vi "Get Speed.vi"(8 "error in (no error)":errorcluster, 11 "Motor in":refnum<class "Motor.lvclass">) -> (0 "error out":errorcluster, 2 "Speed":dbl, 3 "Motor out":refnum<class "Motor.lvclass">)   [LabVIEW 2019, in "Motor.lvclass"]
uses:
  Motor.lvclass
  Motor.lvclass/Motor.ctl
  Motor Serial class/Serial.lvclass
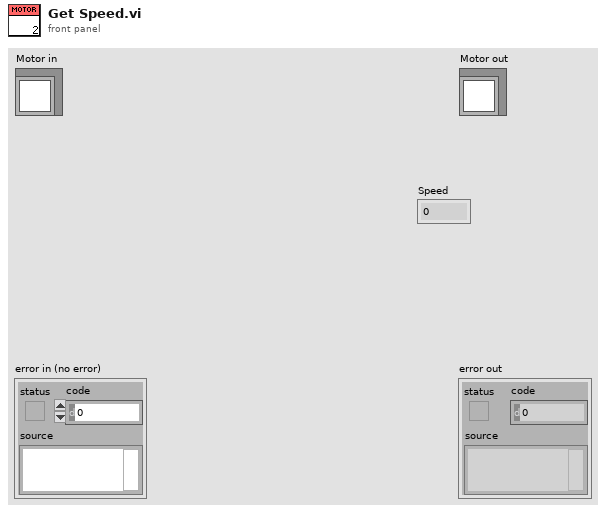
[diagram p1: front panel]
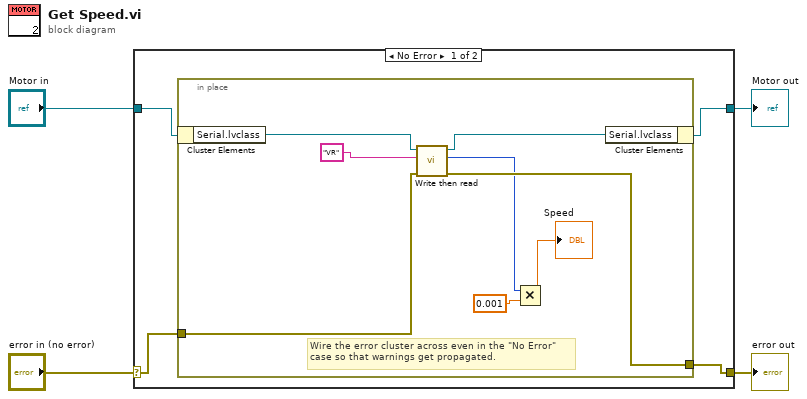
[diagram p0: block diagram]
diagram:
  n1 = case shown="No Error" "error in (no error)" {
    selector: "error in (no error)" -> [w5 w18]
    tunnel: [w6 w18] -> w3
    tunnel: [w7 w17] -> w1
    tunnel: "Motor in" -> [w8 w17]
    frame No Error {
      n2 = in-place {
        in-place-border: [w12] -> w6
        in-place-border: w5 -> [w13]
        # "Wire the error cluster across even in the \"No Error\"\ncase so that warnings get propagated."
        n3 = in-place-cluster #1(w8) -> ("Serial.lvclass"=w16:refnum<class "Serial.lvclass">)
        n4 = call "Write then read.vi"("error in (no error)"=w13, "TX Data"="VR" ("string"), "Motor_Serial in"=w16) -> ("error out"=w12:errorcluster, "RX Data"=w9:i32, "Motor_Serial out"=w15:refnum<class "Serial.lvclass">)  [unwired: 5 in]
        n5 = Multiply(x=w9, y=0.001) -> (x*y=→"Speed":dbl)
        n6 = in-place-cluster #1("Serial.lvclass"=w15) -> (w7:refnum<class "Motor.lvclass">)
      }
    }
    frame Error {
    }
  }
  "error out" <- w3
  "Motor out" <- w1
